vi "PopulatePostProcessing.vi"(6 "Value":refnum<vi>, 9 "Post Processing":refnum<vi>, 10 "PpIndex":refnum<k24>, 11 ".NET Refnum in":refnum<k24>) -> ()   [LabVIEW 2018]
uses:
  D:/SVN/PM/sdk/AppSamples/LabVIEWSamples/trunk/Release/2018/Dependencies/PVCamNET.dll
  Dependencies/PVCamNET.dll
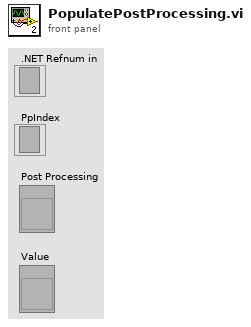
[diagram p1: front panel]
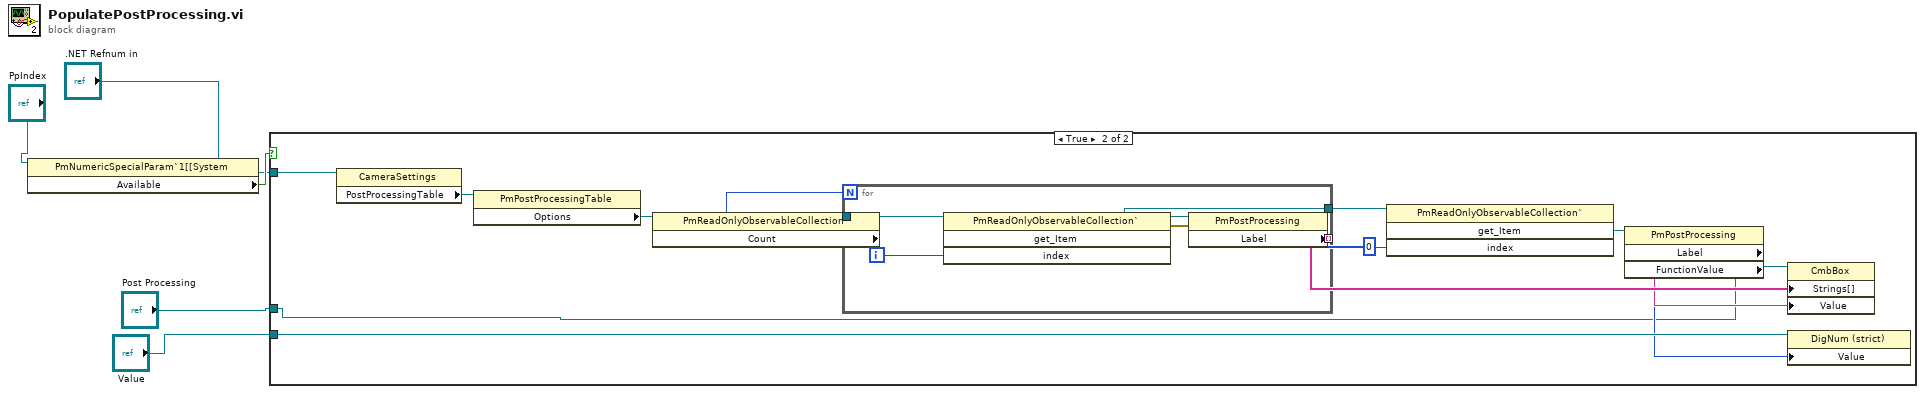
[diagram p0: block diagram]
diagram:
  n1 = property class="PmNumericSpecialParam`1[[System"(reference="PpIndex") -> ("Available"=w4:bool)  [unwired: 1 in, 2 out]
  n2 = case shown="True" w4 {
    tunnel: ".NET Refnum in" -> [_ w18]
    tunnel: "Value" -> [_ w8]
    tunnel: "Post Processing" -> [_ w6]
    frame False {
    }
    frame True {
      n3 = property class="CameraSettings"(reference=w18) -> ("PostProcessingTable"=w17:refnum<k24>)  [unwired: 1 in, 2 out]
      n4 = property class="PmPostProcessingTable"(reference=w17) -> ("Options"=w16:refnum<k24>)  [unwired: 1 in, 2 out]
      n5 = property class="PmReadOnlyObservableCollection`"(reference=w16) -> (reference out=w14:refnum<k24>, "Count"=w15:i32)  [unwired: 1 in, 1 out]
      n6 = for {
        N: w15 -> [_]
        tunnel: w14 -> [w24]
        tunnel: [w21] -> w10 mode=indexing
        tunnel: [w19] -> w13
        i -> [w23]
        n7 = invoke class="PmReadOnlyObservableCollection`" method="get_Item"(reference=w24, "index"=w23) -> (reference out=w19:refnum<k24>, error out=w22:errorcluster, "get_Item"=w20:refnum<k24>)  [unwired: 2 in, 1 out]
        n8 = property class="PmPostProcessing"(reference=w20, error in=w22) -> ("Label"=w21:string)  [unwired: 2 out]
      }
      n9 = invoke class="PmReadOnlyObservableCollection`" method="get_Item"(reference=w13, "index"=0) -> ("get_Item"=w11:refnum<k24>)  [unwired: 2 in, 3 out]
      n10 = property class="PmPostProcessing"(reference=w11) -> ("Label"=w9:string, "FunctionValue"=w7:i32)  [unwired: 1 in, 2 out]
      n11 = property class="CmbBox"(reference=w6, "Strings[]"=w10, "Value"=w9) -> ()  [unwired: 1 in, 2 out]
      n12 = property class="DigNum (strict)"(reference=w8, "Value"=w7) -> ()  [unwired: 1 in, 2 out]
    }
  }
